vi "Convert Transactions to String Arrays.vi"(8 "error in (no error)":errorcluster, 11 "Statement in":refnum<class "TransactionList.lvclass">) -> (0 "error out":errorcluster, 2 "String Arrays":string[](array[string]), 3 "Statement out":refnum<class "TransactionList.lvclass">)   [LabVIEW 2018, in "TransactionList.lvclass"]
uses:
  TransactionList.lvclass
  TransactionList.lvclass/TransactionList.ctl
  Transaction/Transaction.lvclass
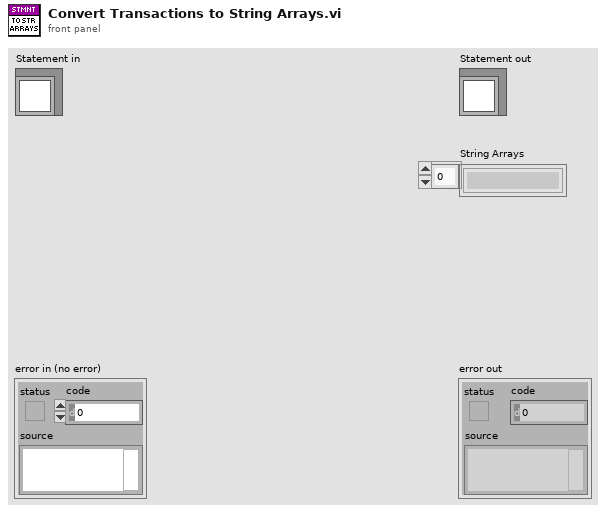
[diagram p1: front panel]
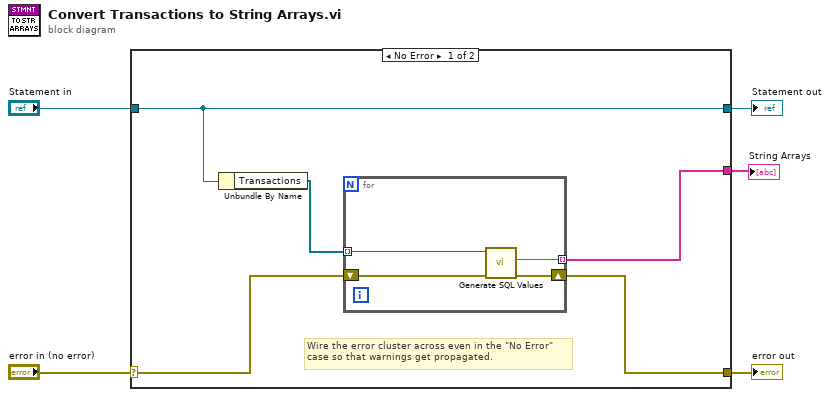
[diagram p0: block diagram]
diagram:
  n1 = case shown="No Error" "error in (no error)" {
    selector: "error in (no error)" -> [w8 w16]
    tunnel: [w7 w16] -> w4
    tunnel: [w10 w15] -> w2
    tunnel: "Statement in" -> [w10 w15]
    tunnel: [w6 _] -> w1
    frame No Error {
      # "Wire the error cluster across even in the \"No Error\"\ncase so that warnings get propagated."
      n2 = Unbundle By Name(w10) -> ("Transactions"=w9:refnum<class "Transaction.lvclass">[])
      n3 = for {
        shift-right: [w14] -> w7
        shift-left: w8 -> [w11]
        tunnel: [w13] -> w6 mode=indexing
        tunnel: w9 -> [w12] mode=indexing
        n4 = call-dynamic "Generate SQL Values.vi"("error in (no error)"=w11, "Transaction in"=w12) -> ("error out"=w14:errorcluster, "SQL Values"=w13:string)  [unwired: 7 in, 1 out]
      }
    }
    frame Error {
    }
  }
  "error out" <- w4
  "Statement out" <- w2
  "String Arrays" <- w1
